vi "I3252_Comm_Interface.vi"(0 "VISA resource name in":refnum<visa-resource-name>, 1 "error in":errorcluster, 5 "Delay (ms)":u32=500, 7 "Write":bool=TRUE, 8 "String to Write":string="*IDN?\n", 10 "Read":bool=TRUE) -> (2 "VISA resource name out":refnum<visa-resource-name>, 3 "error out":errorcluster, 9 "Read String":string)   [LabVIEW 2010]
doc: "The Basic Serial Read and Write example performs a Serial Port Read, a Serial Port Write, or a combination of these actions. The user selects the actions (read or write) on the front panel. If both are selected, the VI will write the data first, read data, and then close the VISA session that is opened to the port. This VI will wait until the specified number of bytes is received at the port or until a termination character is read.\n\nINSTRUCTIONS:\n1) Select the serial resource and configuration parameters (baud rate, data bits, parity, stop bits, flow control).\n2) Select the operations to be performed. \n3) Connect the serial port to your device. If no device is available, perform a loopback test by doing one of the following. Short pins 2 and 3 on a RS-232 cable or short pin 4 to pin 8 and pin 5 to pin 9 on a RS-485/422 cable. \n4) Run the VI to see the data read. (The \"read string\" will match the \"string to write\" if a loopback test was performed.)\n\nNote: The parameters set for the serial port must match the parameters of the connected instrument or device. In this example, the bytes to read parameter specifies the number of bytes that the serial port reads. If there were more bytes at the port than the number specified in bytes to read, those bytes would not be read. Also, if you specify to read more bytes than the number of bytes actually read, you might receive a timeout error message.\n\nOn the block diagram, the Configure Serial Port VI sets the configuration parameters. The front panel displays the controls used to configure the basic parameters, such as baud rate, data bits, and parity. Constants configure the other parameters the user probably does not need set. After the VISA Configure Serial Port VI opens the VISA session and configures the port, the VI passes the VISA resource name to other VIs that perform operations on that VISA resource. The VISA Write function sends a command to the serial device and the VISA Read function returns data based on the command. The VISA Close function then closes the reference to the serial device. It is important to close the reference; otherwise communication through with that port through protocols other than VISA might not be possible."
panel:
  out "Bytes Read":u32
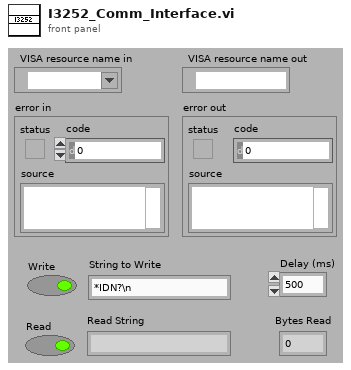
[diagram p1: front panel]
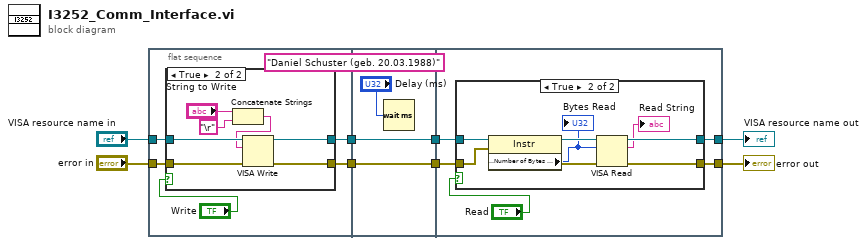
[diagram p0: block diagram]
diagram:
  (unwired) "Daniel Schuster (geb. 20.03.1988)"
  n1 = flat-sequence {
    tunnel: [w12] -> w4
    tunnel: [w13] -> w3
    tunnel: "VISA resource name in" -> [w11]
    tunnel: "error in" -> [w10]
    tunnel: [w24] -> w8
    tunnel: [w23] -> w7
    tunnel: w4 -> [w24]
    tunnel: w3 -> [w23]
    tunnel: w8 -> [w28]
    tunnel: w7 -> [w29]
    tunnel: [w27] -> w6
    tunnel: [w26] -> w5
    frame #0 {
      n2 = case shown="True" "Write" {
        tunnel: [w15 w22] -> w12
        tunnel: w11 -> [w14 w21]
        tunnel: w10 -> [w15 w20]
        tunnel: [w14 w19] -> w13
        frame False {
        }
        frame True {
          n3 = Concatenate Strings("String to Write", "\r") -> (w17:string)
          n4 = VISA Write(VISA resource name=w21, write buffer=w17, error in (no error)=w20) -> (VISA resource name out=w19:refnum<visa-resource-name>, error out=w22:errorcluster)  [unwired: 1 out]
        }
      }
    }
    frame #1 {
      n5 = Wait (ms)(milliseconds to wait="Delay (ms)") -> ()  [unwired: 1 out]
    }
    frame #2 {
      n6 = case shown="True" "Read" {
        tunnel: w28 -> [w32 w36]
        tunnel: [w32 w40] -> w26
        tunnel: [w31 w39] -> w27
        tunnel: w29 -> [w31 w38]
        frame False {
        }
        frame True {
          n7 = property class="Instr"(reference=w38, error in=w36) -> (reference out=w37:refnum<visa-resource-name>, error out=w35:errorcluster, "Serial Settings:Number of Bytes at Serial Port"=w33:u32)
          "Bytes Read" <- w33
          n8 = VISA Read(VISA resource name=w37, byte count=w33, error in (no error)=w35) -> (VISA resource name out=w39:refnum<visa-resource-name>, read buffer=→"Read String":string, error out=w40:errorcluster)  [unwired: 1 out]
        }
      }
    }
  }
  "VISA resource name out" <- w6
  "error out" <- w5
